vi "Remove FPGA Sections.vi"(8 "error in (no error)":errorcluster, 11 "Item Ref in":T1 format="%.0x") -> (0 "error out":errorcluster, 3 "Item Ref out":T1 format="%.0x")   [LabVIEW 2019, in "FPGA Addon System Explorer.lvlib"]
uses:
  FPGA Addon System Explorer.lvlib
  <vilib>/NI VeriStand/Custom Device API/Custom Device Item Ref.ctl
  <vilib>/NI VeriStand/Custom Device API/Custom Device API.lvlib
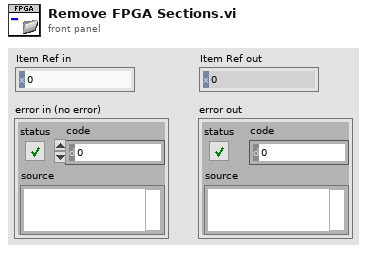
[diagram p1: front panel]
types:
  T1 = typedef "Custom Device API.lvlib/Custom Device Item Ref.ctl" = u64
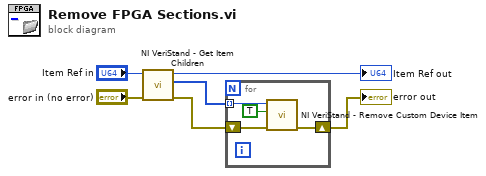
[diagram p0: block diagram]
diagram:
  n1 = call <vilib>:"NI VeriStand - Get Item Children.vi"("error in (no error)"="error in (no error)", "Item Ref in"="Item Ref in") -> ("error out"=w2:errorcluster, "Child Refs"=w1:T1[], "Item Ref out"=→"Item Ref out":T1)  [unwired: 6 in, 1 out]
  n2 = for {
    tunnel: w1 -> [w10] mode=indexing
    shift-right: [w8] -> w6
    shift-left: w2 -> [w9]
    n3 = call <vilib>:"NI VeriStand - Remove Custom Device Item.vi"("error in (no error)"=w9, "Force Delete (F)"=TRUE, "Item Ref in"=w10) -> ("error out"=w8:errorcluster)  [unwired: 7 in, 1 out]
  }
  "error out" <- w6
